vi "消息推送core.vi"(8 "error in (no error)":errorcluster caption="错误输入（无错误）", 10 "数组":string[](array[string])=["UID_u2gUaG5SHjMBZfWcukaJD0Ypef0K"], 11 "content":string) -> (0 "error out":errorcluster caption="错误输出", 3 "GBK":string)   [LabVIEW 2016, in "Alarm interface.lvlib" / "wxpusher.lvlib"]
uses:
  wxpusher.lvlib
  <vilib>/httpClient/POSTBuffer.vi
  <vilib>/httpClient/LabVIEWHTTPClient.lvlib
panel:
  out "JSON字符串":string
  out "headers":string caption="头部"
  out "body":string caption="体部"
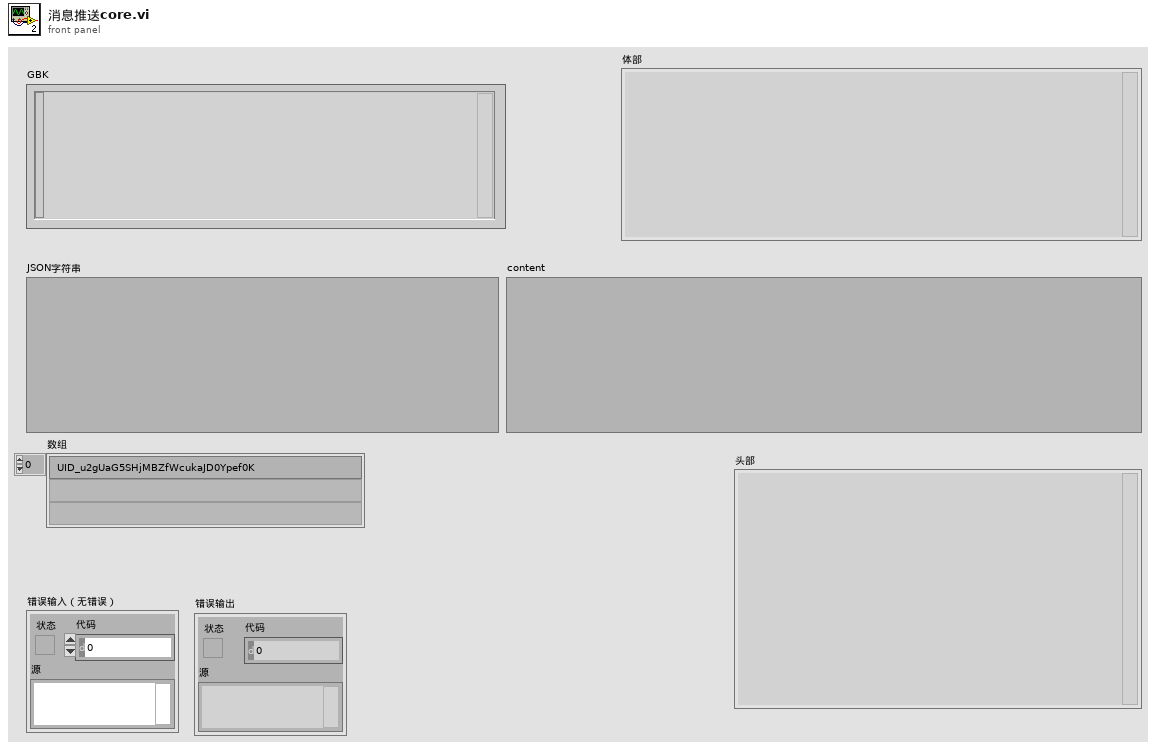
[diagram p1: front panel]
types:
  T1 = cluster{"code":i32, "msg":string, "data":cluster{"uid":string, "topicId":ext, "messageId":ext, "code":ext, "status":string}[], "success":bool}
  T2 = cluster{"appToken":string, "content":string, "contentType":i32, "topicIds":i32[], "uids":string[], "url":string}
  T3 = enum16{"open", "replace", "create", "open or create", "replace or create", "replace or create with confirmation"}
  T4 = typedef "LabVIEWHTTPClient.lvlib/ClientHandle.ctl" = refnum<k1>
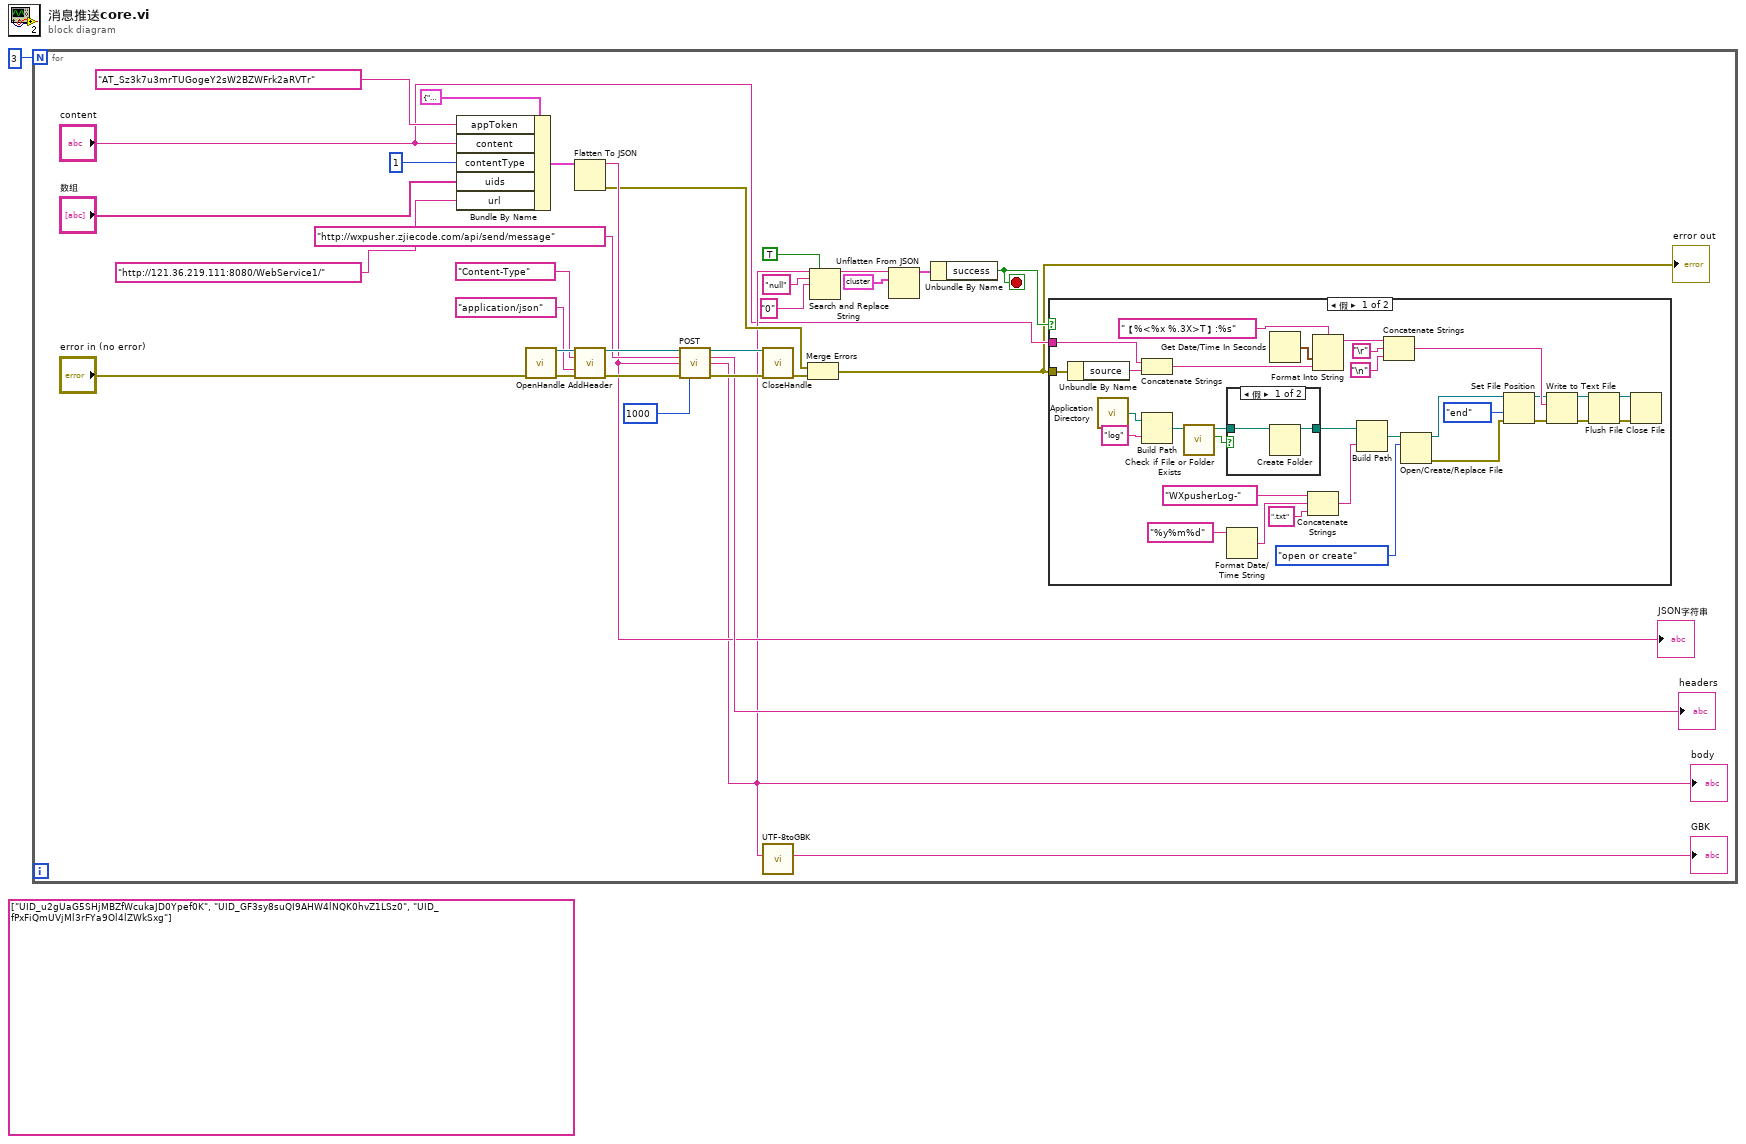
[diagram p0: block diagram]
diagram:
  (unwired) string[] ["UID_u2gUaG5SHjMBZfWcukaJD0Ypef0K", "UID_GF3sy8suQI9AHW4lNQK0hvZ1LSz0", "UID_fPxFiQmUVjMl3rFYa9Ol4lZWkSxg"]
  n1 = for {
    N: 3 -> [_]
    stop <- w4 stop-if-true
    n2 = Bundle By Name(cluster=T2 {"appToken"="", "content"="", "contentType"=0, "topicIds"=[], "uids"=[], "url"=""}, "appToken"="AT_Sz3k7u3mrTUGogeY2sW2BZWFrk2aRVTr", "content"="content", "contentType"=1, "uids"="数组", "url"="http://121.36.219.111:8080/WebService1/" ("输入 5")) -> (w20:T2)
    n3 = call <vilib>:"OpenHandle.vi"("error in (no error)"="error in (no error)") -> ("client handle out"=w33:T4, "error out"=w31:errorcluster)  [unwired: 13 in]
    n4 = Flatten To JSON(anything=w20) -> (JSON string=w19:string, 11:w12:errorcluster)  [unwired: 2 in]
    "JSON字符串" <- w19
    n5 = call <vilib>:"AddHeader.vi"("client handle"=w33, "header"="Content-Type", "value"="application/json", "error in (no error)"=w31) -> ("client handle out"=w32:T4, "error out"=w28:errorcluster)  [unwired: 10 in]
    n6 = call-poly <vilib>:"POST.vi"("client handle"=w32, "url"="http://wxpusher.zjiecode.com/api/send/message", "buffer"=w19, "error in (no error)"=w28, "timeout (10000)"=1000) -> ("client handle out"=w25:T4, "headers"=→"headers":string, "body"=w6:string, "error out"=w26:errorcluster)  [unwired: 7 in]
    "body" <- w6
    n7 = call <vilib>:"CloseHandle.vi"("client handle"=w25, "error in (no error)"=w26) -> ("error out"=w13:errorcluster)  [unwired: 13 in]
    n8 = call "UTF-8toGBK.vi"("UTF-8"=w6) -> ("GBK"=→"GBK":string)  [unwired: 9 in, 1 out]
    n9 = Merge Errors(w12, w13) -> (w2:errorcluster)
    "error out" <- w2
    n10 = Search and Replace String(replace all?=TRUE ("替换全部？(F)"), input string=w6, search string="null" ("搜索字符串"), replace string="0" ("替换字符串(\"\")")) -> (result string=w7:string)  [unwired: 4 in, 3 out]
    n11 = Unflatten From JSON(JSON string=w7, type and defaults=T1 {"code"=0, "msg"="", "data"=[{"uid"="", "topicId"=0.0, "messageId"=0.0, "code"=0.0, "status"=""}], "success"=TRUE}) -> (value=w5:T1)  [unwired: 5 in, 1 out]
    n12 = Unbundle By Name(w5) -> ("success"=w4:bool)
    n13 = case shown="假" w4 {
      tunnel: "content" -> [w36 _]
      tunnel: w2 -> [w37 _]
      frame False {
        n14 = Unbundle By Name(w37) -> ("source"=w35:string)
        n15 = call <vilib>:"Application Directory.vi"() -> ("Application Directory"=w59:path)
        n16 = Concatenate Strings(w36, w35) -> (w34:string)
        n17 = Build Path(base path=w59, name or relative path="log" ("名称或相对路径")) -> (appended path=w61:path)
        n18 = call <vilib>:"Check if File or Folder Exists.vi"("path"=w61) -> ("file or folder exists?"=w46:bool, "dup path"=w47:path)  [unwired: 8 in, 1 out]
        n19 = case shown="假" w46 {
          tunnel: w47 -> [w67 w68]
          tunnel: [w66 w68] -> w48
          frame False {
            n20 = Create Folder(path (use dialog)=w67) -> (created path=w66:path)  [unwired: 2 in, 2 out]
          }
          frame True {
          }
        }
        n21 = Format Date/Time String(time format string (%c)="%y%m%d" ("时间格式字符串(%c)")) -> (date/time string=w50:string)  [unwired: 2 in]
        n22 = Get Date/Time In Seconds() -> (seconds since 1Jan1904=w39:timestamp)
        n23 = Concatenate Strings("WXpusherLog-" ("字符串"), w50, ".txt" ("字符串")) -> (w51:string)
        n24 = Format Into String(format string="【%<%x %.3X>T】:%s" ("格式字符串"), w39, w34) -> (resulting string=w40:string)  [unwired: 2 in, 1 out]
        n25 = Build Path(base path=w48, name or relative path=w51) -> (appended path=w52:path)
        n26 = Concatenate Strings(w40, "\r", "\n") -> (w63:string)
        n27 = Open/Create/Replace File(file path (use dialog)=w52, operation (0:open)=T3."open or create" ("操作(0:open)")) -> (refnum out=w44:refnum<file>, error out=w42:errorcluster)  [unwired: 4 in, 1 out]
        n28 = Set File Position(refnum=w44, from (0:start)=enum16{"start", "end", "current"}."end" ("自（0:起始）"), error in=w42) -> (refnum out=w43:refnum<file>, error out=w41:errorcluster)  [unwired: 1 in]
        n29 = Write to Text File(file (use dialog)=w43, text=w63, error in=w41) -> (refnum out=w56:refnum<file>, error out=w57:errorcluster)  [unwired: 1 in, 1 out]
        n30 = Flush File(refnum=w56, error in=w57) -> (refnum out=w54:refnum<file>, error out=w55:errorcluster)
        n31 = Close File(refnum=w54, error in=w55) -> ()  [unwired: 2 out]
      }
      frame True {
      }
    }
  }
